vi "Example 2.vi"   [LabVIEW 2018]
uses:
  <vilib>/addons/VeriStand Custom Device Scripting APIs/FPGA Addon/Scripting API.lvlib
  <vilib>/addons/VeriStand Custom Device Scripting APIs/FPGA Addon/TypeDefs/Input Scalar Data.ctl
  <vilib>/addons/VeriStand Custom Device Scripting APIs/FPGA Addon/Private/Import Bitfile Scalars (Instances)/Import Scalars - by label.vi
types:
  T1 = typedef "Scripting API.lvlib/Input Scalar Data.ctl" = cluster{"Bitfile Name":string, "SysDef Name":string}
  T2 = typedef "Custom Device API.lvlib/Custom Device Item Ref.ctl" = u64
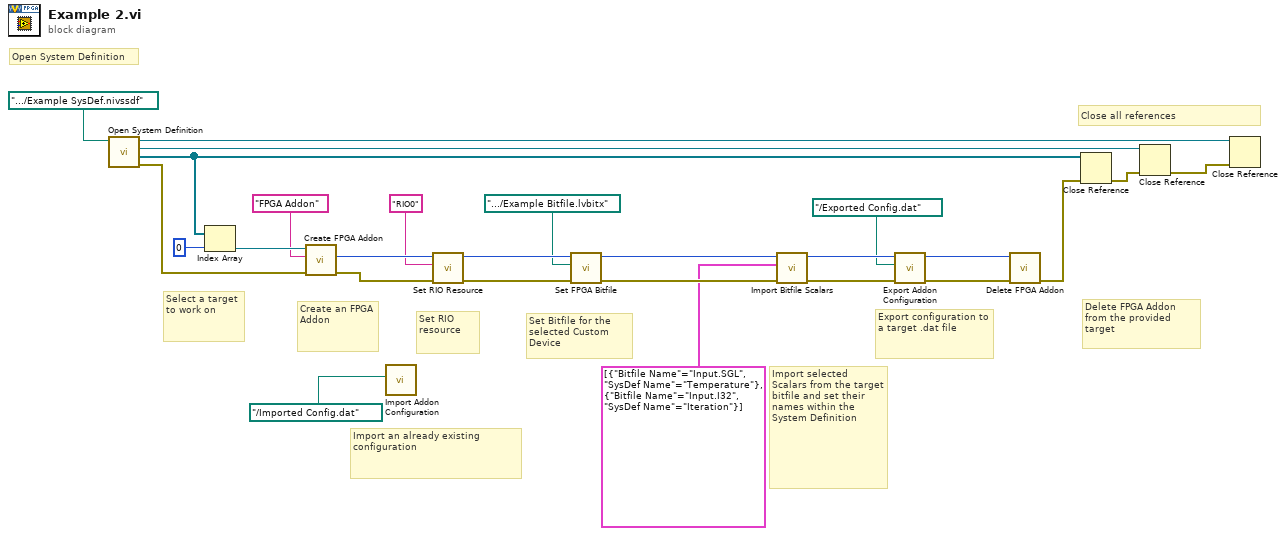
[diagram p0: block diagram]
diagram:
  # "Delete FPGA Addon from the provided target"
  # "Export configuration to a target .dat file"
  # "Import an already existing configuration"
  # "Import selected Scalars from the target bitfile and set their names within the System Definition"
  # "Close all references"
  # "Set Bitfile for the selected Custom Device"
  # "Set RIO resource"
  # "Create an FPGA Addon"
  # "Select a target to work on"
  # "Open System Definition"
  n1 = call <vilib>:"Open System Definition.vi"("System Definition File"=path ".../Example SysDef.nivssdf" ("fpga bitfile path")) -> ("error out"=w23:errorcluster, "targets refnums"=w11:refnum<k24>[], "root refnum"=w12:refnum<k24>, "system definition refnum"=w13:refnum<k24>)  [unwired: 7 in]
  n2 = Index Array(array=w11, index=0) -> (element=w25:refnum<k24>)
  n3 = call <vilib>:"Create FPGA Addon.vi"("error in (no error)"=w23, "fpga addon name"="FPGA Addon", "target in"=w25) -> ("error out"=w21:errorcluster, "fpga addon refnum"=w22:T2)  [unwired: 6 in, 1 out]
  n4 = call <vilib>:"Import Addon Configuration.vi"("configuration file path"=path "../Imported Config.dat" ("export file path")) -> ()  [unwired: 9 in, 2 out]
  n5 = call <vilib>:"Set RIO Resource.vi"("error in (no error)"=w21, "rio resource in"="RIO0", "fpga addon refnum in"=w22) -> ("error out"=w19:errorcluster, "fpga addon refnum out"=w18:T2)  [unwired: 7 in]
  n6 = call <vilib>:"Set FPGA Bitfile.vi"("error in (no error)"=w19, "fpga bitfile path"=path ".../Example Bitfile.lvbitx", "fpga addon refnum in"=w18) -> ("error out"=w15:errorcluster, "fpga addon refnum out"=w14:T2)  [unwired: 7 in]
  n7 = call-poly <vilib>:"Import Bitfile Scalars.vi"("error in (no error)"=w15, "bitfile scalars in"=T1[] [{"Bitfile Name"="Input.SGL", "SysDef Name"="Temperature"}, {"Bitfile Name"="Input.I32", "SysDef Name"="Iteration"}], "fpga addon refnum in"=w14) -> ("error out"=w7:errorcluster, "fpga addon refnum out"=w6:T2)  [unwired: 6 in, 1 out]
  n8 = call <vilib>:"Export Addon Configuration.vi"("error in (no error)"=w7, "export file path"=path "../Exported Config.dat", "fpga addon refnum in"=w6) -> ("error out"=w3:errorcluster, "fpga addon refnum out"=w2:T2)  [unwired: 7 in]
  n9 = call <vilib>:"Delete FPGA Addon.vi"("error in (no error)"=w3, "fpga addon refnum"=w2) -> ("error out"=w1:errorcluster)  [unwired: 9 in]
  n10 = Close Reference(reference=w11, error in (no error)=w1) -> (error out=w10:errorcluster)
  n11 = Close Reference(reference=w12, error in (no error)=w10) -> (error out=w9:errorcluster)
  n12 = Close Reference(reference=w13, error in (no error)=w9) -> ()  [unwired: 1 out]
